vi "CleanDependencies.vi"(8 "error in (no error)":errorcluster, 10 "Dependency":refnum<class "SMO.lvclass">, 11 "SMO in":refnum<class "SMO.lvclass">) -> (0 "error out":errorcluster, 3 "SMO out":refnum<class "SMO.lvclass">, 4 "Removed":bool)   [LabVIEW 2013, in "SMO.lvclass"]
uses:
  SMO.lvclass
  SMO.lvclass/SMO.ctl
  ReftoDVR--SMO.vi
  Support/Attribute.Dependencies/Attribute.Dependencies.lvclass
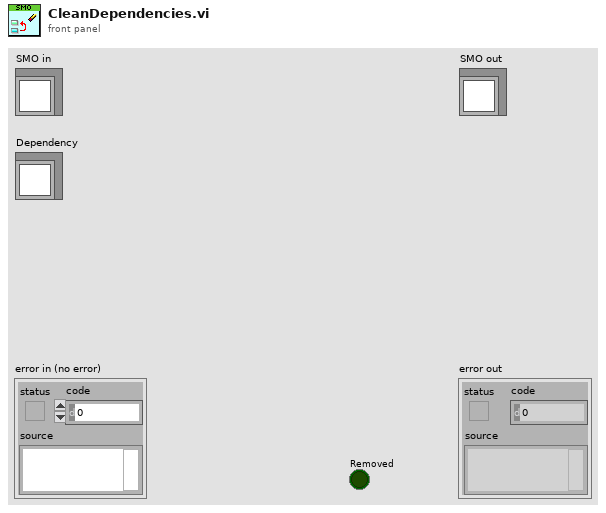
[diagram p1: front panel]
types:
  T1 = typedef "Attribute.Dependencies.lvclass/DependencyAttr--Cluster.ctl" = cluster{"Name":string, "GUID":string, "owned":bool, "shared":bool, "Level":string, "SMO":refnum<class "SMO.lvclass">}
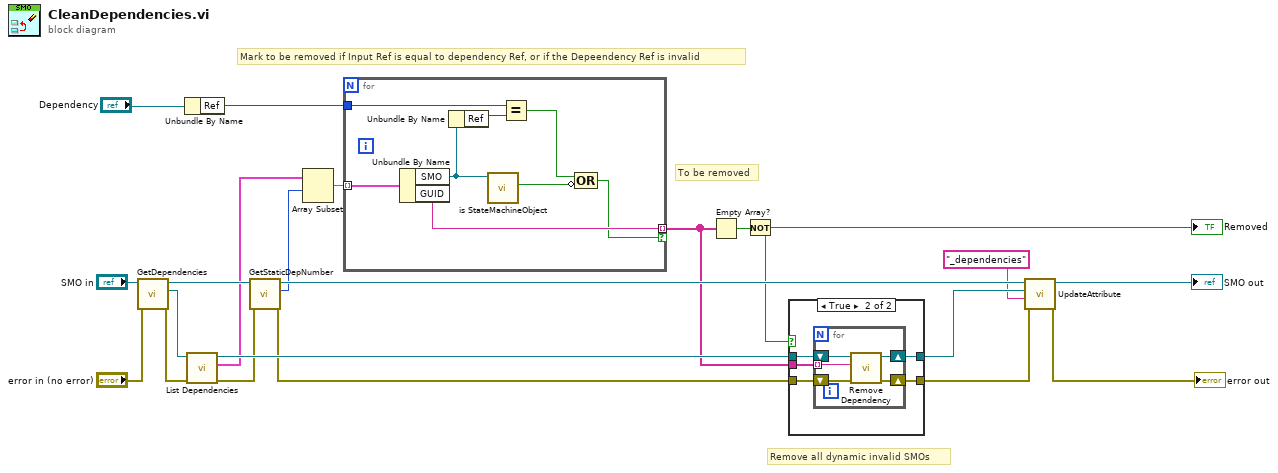
[diagram p0: block diagram]
diagram:
  # "Mark to be removed if Input Ref is equal to dependency Ref, or if the Depeendency Ref is invalid"
  # "To be removed"
  # "Remove all dynamic invalid SMOs"
  n1 = call "GetDependencies.vi"("error in (no error)"="error in (no error)", "SMO in"="SMO in") -> ("error out"=w17:errorcluster, "Dependencies"=w20:refnum<class "Attribute.Dependencies.lvclass">, "SMO out"=w16:refnum<class "SMO.lvclass">)  [unwired: 7 in]
  n2 = Unbundle By Name("Dependency") -> ("Ref"=w21:u32)
  n3 = call "List Dependencies.vi"("error in (no error)"=w17, "Attribute.Dependencies in"=w20) -> ("error out"=w6:errorcluster, "Dependencies"=w3:T1[], "Attribute.Dependencies out"=w9:refnum<class "Attribute.Dependencies.lvclass">)  [unwired: 7 in]
  n4 = call "GetStaticDepNumber.vi"("error in (no error)"=w6, "SMO in"=w16) -> ("error out"=w5:errorcluster, "Nb of Static Dependencies"=w4:u32, "SMO out"=w14:refnum<class "SMO.lvclass">)  [unwired: 7 in]
  n5 = Array Subset(array=w3, index=w4) -> (w2:T1[])  [unwired: 1 in]
  n6 = for {
    tunnel: [w25] -> w7 mode=indexing if=w23
    tunnel: w21 -> [w29]
    tunnel: w2 -> [w26] mode=indexing
    n7 = Unbundle By Name(w26) -> ("SMO"=w30:refnum<class "SMO.lvclass">, "GUID"=w25:string)
    n8 = Unbundle By Name(w30) -> ("Ref"=w28:u32)
    n9 = call "is StateMachineObject.vi"("SMO"=w30) -> ("is SMO?"=w24:bool)  [unwired: 8 in, 2 out]
    n10 = Equal?(x=w29, y=w28) -> (x = y?=w27:bool)
    n11 = Compound Arithmetic op=OR(w27, invert w24) -> (w23:bool)
  }
  n12 = Empty Array?(array=w7) -> (empty?=w15:bool)
  n13 = Not(x=w15) -> (.not. x?=w8:bool)
  "Removed" <- w8
  n14 = case shown="True" w8 {
    tunnel: [w32 w37] -> w12
    tunnel: [w31 w36] -> w10
    tunnel: w5 -> [w31 w35]
    tunnel: w9 -> [w32 w34]
    tunnel: w7 -> [_ w33]
    frame False {
    }
    frame True {
      n15 = for {
        shift-right: [w42] -> w37
        shift-left: w34 -> [w40]
        shift-right: [w41] -> w36
        shift-left: w35 -> [w39]
        tunnel: w33 -> [w38] mode=indexing
        n16 = call "Remove Dependency.vi"("error in (no error)"=w39, "GUID"=w38, "Attribute.Dependencies in"=w40) -> ("error out"=w41:errorcluster, "Attribute.Dependencies out"=w42:refnum<class "Attribute.Dependencies.lvclass">)  [unwired: 7 in]
      }
    }
  }
  n17 = call "UpdateAttribute.vi"("error in (no error)"=w10, "Attribute Name"="_dependencies", "Attribute"=w12, "SMO in"=w14) -> ("error out"=→"error out":errorcluster, "SMO out"=→"SMO out":refnum<class "SMO.lvclass">)  [unwired: 5 in, 1 out]
